vi "Main Page.vi"(8 "error in (no error)":errorcluster, 11 "Node Ptr":T1 format="%.0x") -> (0 "error out":errorcluster)   [LabVIEW 2015, in "FPGA Addon System Explorer.lvlib"]
uses:
  FPGA Addon System Explorer.lvlib
  <vilib>/NI Veristand/Custom Device API/Custom Device Item Ref.ctl
  Shared/FG Action.ctl
  Shared/Constants.vi
  <vilib>/NI Veristand/Custom Device API/NI VeriStand - Get Item Property.vi
  <vilib>/NI Veristand/Custom Device API/Get Item Property (Path).vi
  <vilib>/NI Veristand/Custom Device API/Get Item Property (String).vi
  <vilib>/NI Veristand/Custom Device API/NI VeriStand - Set Item Property.vi
  <vilib>/NI Veristand/Custom Device API/Set Item Property (Path).vi
  <vilib>/NI Veristand/Custom Device API/Set Item Property (String).vi
  <vilib>/NI VeriStand/Custom Device API/Custom Device API.lvlib
  Shared/FPGA Addon Shared.lvlib
panel:
  out "Version":string
  in  "SHDocVw.IWebBrowser":refnum<k7>(container)
  in  "RIO Device Address":string
  in  "Bitfile path":path
  in  "Header 2":cluster{"Section Name":string}={"Section Name"="Custom Device Item Settings"}
  in  "Header":cluster{"Section Name":string}={"Section Name"="Custom Device Item Settings"}
  in  "Description":string
  in  "Name":string
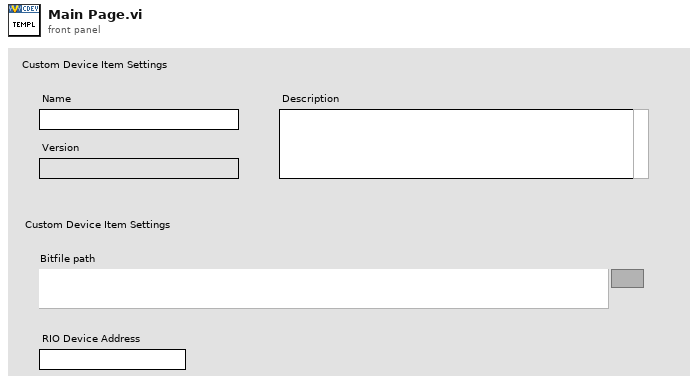
[diagram p1: front panel]
types:
  T1 = typedef "Custom Device API.lvlib/Custom Device Item Ref.ctl" = u64
  T2 = typedef "FPGA Addon Shared.lvlib/FG Action.ctl" = enum8{"GET", "SET"}
  T3 = typedef "FPGA Addon Shared.lvlib/FPGA Settings.ctl" = cluster{"Bitfile path":path, "RIO Device Address":string}
  T4 = typedef "Custom Device API.lvlib/Custom Device Item Info.ctl" = cluster{"Name":string, "Is Channel":bool, "GUID":string, "Is Waveform":bool}
  T5 = typedef "Custom Device API.lvlib/Custom Device Commands.ctl" = enum16{"Default", "Item renamed", "Shutdown", "Dynamic button pressed"}
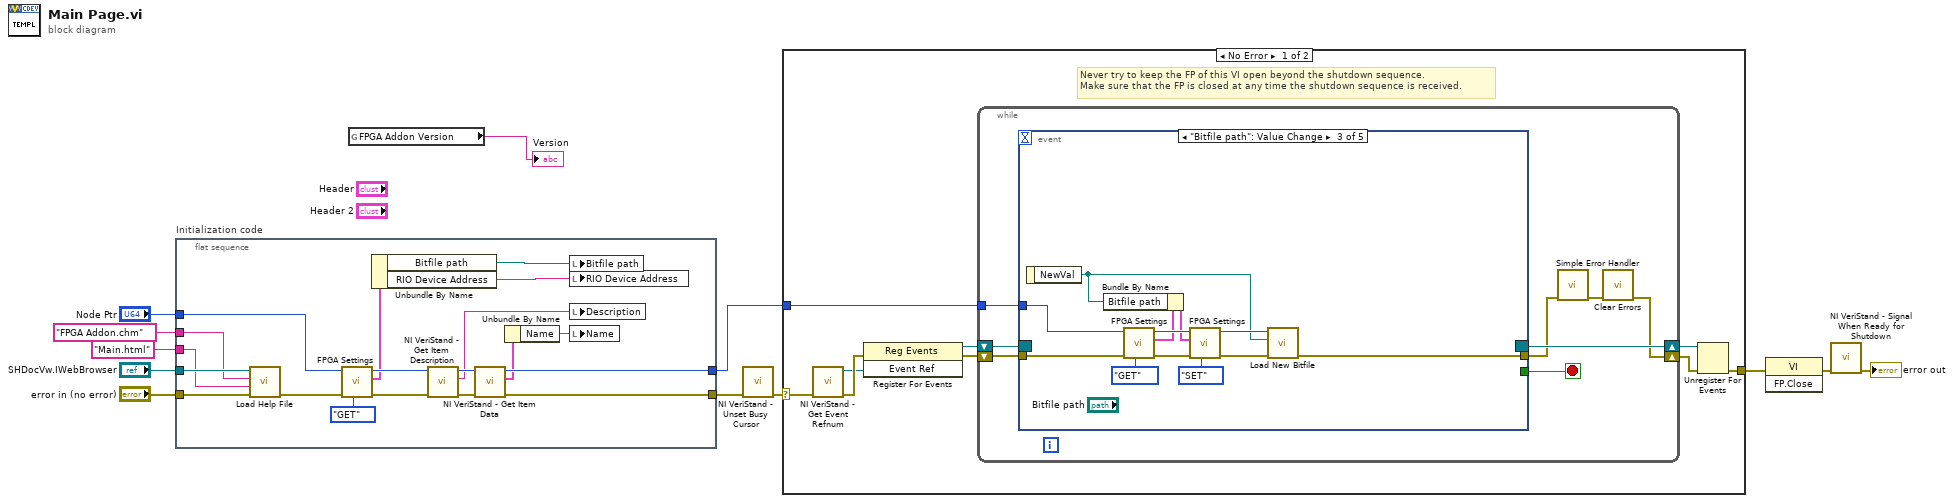
[diagram p0: block diagram]
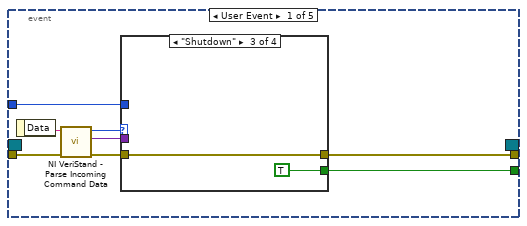
[diagram p2: hidden frame]
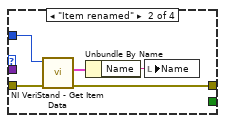
[diagram p4: hidden frame]
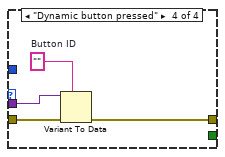
[diagram p5: hidden frame]
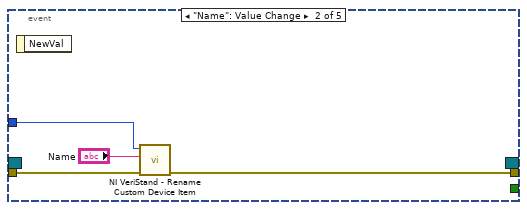
[diagram p6: hidden frame]
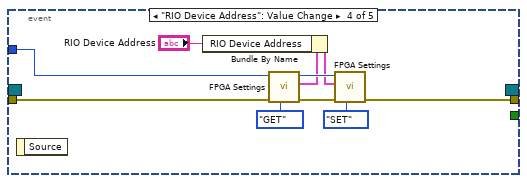
[diagram p7: hidden frame]
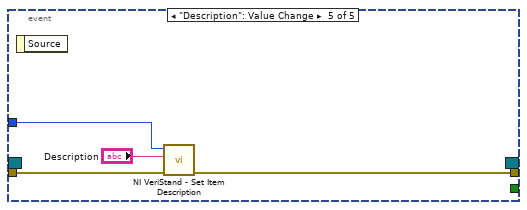
[diagram p8: hidden frame]
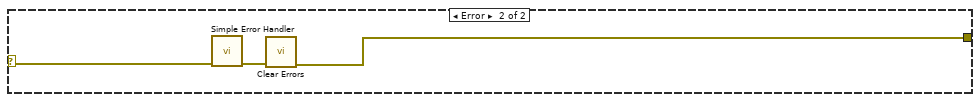
[diagram p9: hidden frame]
diagram:
  n1 = flat-sequence "Initialization code" {
    tunnel: "error in (no error)" -> [w24]
    tunnel: "Node Ptr" -> [w20]
    tunnel: [w25] -> w8
    tunnel: [w31] -> w5
    tunnel: "SHDocVw.IWebBrowser" -> [w23]
    tunnel: "Main.html" ("HTML File") -> [w22]
    tunnel: "FPGA Addon.chm" ("Main CHM File") -> [w21]
    frame #0 {
      n2 = call "Load Help File.vi"("error in (no error)"=w24, "HTML File"=w22, "Main CHM File"=w21, "SHDocVw.IWebBrowser2"=w23) -> ("error out"=w19:errorcluster)  [unwired: 7 in]
      n3 = call "FPGA Settings.vi"("Action"=FG_Action."GET", "error in (no error)"=w19, "Item Ref"=w20) -> ("error out"=w17:errorcluster, "FPGA Settings"=w15:T3, "Item Ref out"=w18:T1)  [unwired: 6 in]
      n4 = Unbundle By Name(w15) -> ("Bitfile path"=w13:path, "RIO Device Address"=w14:string)
      n5 = call <vilib>:"NI VeriStand - Get Item Description.vi"("error in (no error)"=w17, "Item Ref in"=w18) -> ("error out"=w28:errorcluster, "Description"=w29:string, "Item Ref out"=w30:T1)  [unwired: 7 out]
      n6 = call <vilib>:"NI VeriStand - Get Item Data.vi"("error in (no error)"=w28, "Item Ref in"=w30) -> ("error out"=w25:errorcluster, "Item Info"=w27:T4, "Item Ref out"=w31:T1)  [unwired: 7 out]
      n7 = Unbundle By Name(w27) -> ("Name"=w26:string)
      n8 = local write "Bitfile path"(w13) -> ()
      n9 = local write "RIO Device Address"(w14) -> ()
      n10 = local write "Description"(w29) -> ()
      n11 = local write "Name"(w26) -> ()
    }
  }
  n12 = global read "Constants.vi" "FPGA Addon Version"() -> (→"Version":string)
  n13 = call <vilib>:"NI VeriStand - Unset Busy Cursor.vi"("error in (no error)"=w8) -> ("error out"=w7:errorcluster)  [unwired: 10 out]
  n14 = case shown="No Error" w7 {
    selector: w7 -> [w32 w101]
    tunnel: [w37 w99] -> w12
    tunnel: w5 -> [w33 _]
    frame No Error {
      # "Never try to keep the FP of this VI open beyond the shutdown sequence.\nMake sure that the FP is closed at any time the shutdown sequence is received."
      n15 = call <vilib>:"NI VeriStand - Get Event Refnum.vi"("error in (no error)"=w32) -> ("error out"=w40:errorcluster, "Event Ref"=w36:refnum<user-event>)  [unwired: 9 out]
      n16 = register-events(error in=w40, w36) -> (reference out=w34:refnum<event-registration>, error out=w35:errorcluster)  [unwired: 1 in]
      n17 = while {
        tunnel: w33 -> [w44]
        shift-right: [w41] -> w38
        shift-left: w35 -> [w47]
        shift-right: [w48] -> w39
        shift-left: w34 -> [w46]
        stop <- w45 stop-if-true
        n18 = event shown="[2] \"Bitfile path\": Value Change" {
          selector: w46 -> [_ _ _ _ _]
          dyn-events: [_ _ _ _ _] -> w48
          timeout: _ -> [_ _ _ _ _]
          tunnel: w47 -> [w56 w72 w79 w88 w97]
          tunnel: [w52 _ _ _ _] -> w45
          tunnel: [w51 w71 w84 w85 w96] -> w43
          tunnel: w44 -> [w50 w70 w77 w87 w98]
          event User Event {
            n19 = event-data() -> ("Data"=w55:string)  [unwired: 1 out]
            n20 = call <vilib>:"NI VeriStand - Parse Incoming Command Data.vi"("error in (no error)"=w56, "Incoming data"=w55) -> ("error out"=w54:errorcluster, "Outgoing data"=w49:variant, "Action"=w53:T5)  [unwired: 7 out]
            n21 = case shown="\"Shutdown\"" w53 {
              tunnel: w54 -> [w57 w62 w63 w68]
              tunnel: [_ _ TRUE _] -> w52
              tunnel: [w57 w59 w63 w65] -> w51
              tunnel: w50 -> [_ w61 _ _]
              tunnel: w49 -> [_ _ _ w67]
              frame "Default", Default {
              }
              frame "Item renamed" {
                n22 = call <vilib>:"NI VeriStand - Get Item Data.vi"("error in (no error)"=w62, "Item Ref in"=w61) -> ("error out"=w59:errorcluster, "Item Info"=w60:T4)  [unwired: 8 out]
                n23 = Unbundle By Name(w60) -> ("Name"=w58:string)
                n24 = local write "Name"(w58) -> ()
              }
              frame "Shutdown" {
              }
              frame "Dynamic button pressed" {
                w66 = ""  # Button ID
                n25 = Variant To Data(error in=w68, type=w66, Variant=w67) -> (error out=w65:errorcluster)  [unwired: 1 out]
              }
            }
          }
          event "Name": Value Change {
            n26 = event-data() -> ()  [unwired: 2 out]
            n27 = call <vilib>:"NI VeriStand - Rename Custom Device Item.vi"("error in (no error)"=w72, "New Name"="Name", "Item Ref in"=w70) -> ("error out"=w71:errorcluster)  [unwired: 1 in, 7 out]
          }
          event "Bitfile path": Value Change {
            n28 = event-data() -> ("NewVal"=w73:path)  [unwired: 1 out]
            n29 = call "FPGA Settings.vi"("Action"=FG_Action."GET", "error in (no error)"=w79, "Item Ref"=w77) -> ("error out"=w80:errorcluster, "FPGA Settings"=w75:T3, "Item Ref out"=w81:T1)  [unwired: 6 in]
            n30 = Bundle By Name(cluster=w75, "Bitfile path"=w73) -> (w74:T3)
            n31 = call "FPGA Settings.vi"("Action"=FG_Action."SET", "error in (no error)"=w80, "FPGA Settings"=w74, "Item Ref"=w81) -> ("error out"=w78:errorcluster, "Item Ref out"=w76:T1)  [unwired: 5 in, 1 out]
            n32 = call "Load New Bitfile.vi"("error in (no error)"=w78, "NewVal"=w73, "Item Ref in"=w76) -> ("error out"=w84:errorcluster)  [unwired: 7 in, 1 out]
          }
          event "RIO Device Address": Value Change {
            n33 = event-data() -> ()  [unwired: 2 out]
            n34 = call "FPGA Settings.vi"("Action"=FG_Action."GET", "error in (no error)"=w88, "Item Ref"=w87) -> ("error out"=w91:errorcluster, "FPGA Settings"=w90:T3, "Item Ref out"=w92:T1)  [unwired: 6 in]
            n35 = Bundle By Name(cluster=w90, "RIO Device Address"="RIO Device Address") -> (w89:T3)
            n36 = call "FPGA Settings.vi"("Action"=FG_Action."SET", "error in (no error)"=w91, "FPGA Settings"=w89, "Item Ref"=w92) -> ("error out"=w85:errorcluster)  [unwired: 5 in, 2 out]
          }
          event "Description": Value Change {
            n37 = event-data() -> ()  [unwired: 2 out]
            n38 = call <vilib>:"NI VeriStand - Set Item Description.vi"("error in (no error)"=w97, "Description"="Description", "Item Ref in"=w98) -> ("error out"=w96:errorcluster)  [unwired: 8 out]
          }
        }
        n39 = call <vilib>:"Simple Error Handler.vi"("error in (no error)"=w43) -> ("error out"=w42:errorcluster)  [unwired: 1 in, 7 out]
        n40 = call <vilib>:"Clear Errors.vi"("error in (no error)"=w42) -> ("error out"=w41:errorcluster)  [unwired: 1 in, 5 out]
      }
      n41 = Unregister For Events(event registration refnum=w39, error in=w38) -> (error out=w37:errorcluster)
    }
    frame Error {
      n42 = call <vilib>:"Simple Error Handler.vi"("error in (no error)"=w101) -> ("error out"=w100:errorcluster)  [unwired: 1 in, 7 out]
      n43 = call <vilib>:"Clear Errors.vi"("error in (no error)"=w100) -> ("error out"=w99:errorcluster)  [unwired: 1 in, 5 out]
    }
  }
  n44 = invoke class="VI" method="FP.Close"(error in=w12) -> (error out=w11:errorcluster)  [unwired: 2 in, 2 out]
  n45 = call <vilib>:"NI VeriStand - Signal When Ready for Shutdown.vi"("error in (no error)"=w11) -> ("error out"=→"error out":errorcluster)  [unwired: 10 out]
